vi "GHV232 CRAB Error Message.vi"(11 "Receive Packet":string) -> (0 "Message":string)   [LabVIEW 2017]
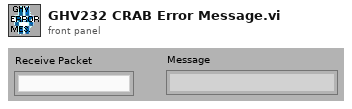
[diagram p1: front panel]
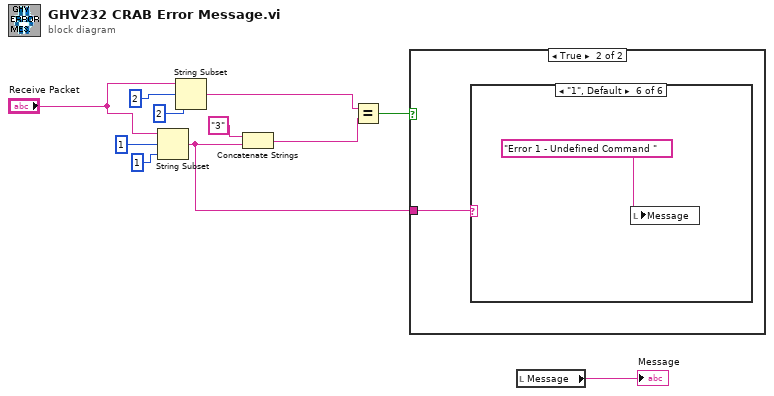
[diagram p0: block diagram]
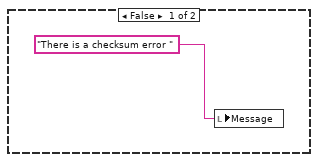
[diagram p2: hidden frame]
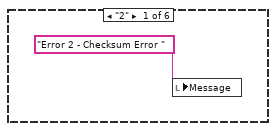
[diagram p3: hidden frame]
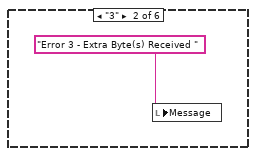
[diagram p4: hidden frame]
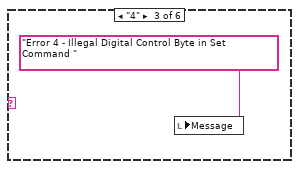
[diagram p5: hidden frame]
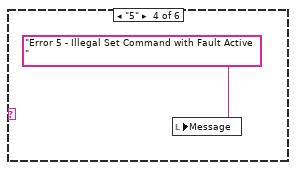
[diagram p6: hidden frame]
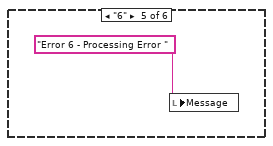
[diagram p7: hidden frame]
diagram:
  n1 = String Subset(string="Receive Packet", offset (0)=1, length (rest)=1) -> (substring=w5:string)
  n2 = String Subset(string="Receive Packet", offset (0)=2, length (rest)=2) -> (substring=w3:string)
  n3 = Concatenate Strings("3", w5) -> (w2:string)
  n4 = Equal?(x=w3, y=w2) -> (x = y?=w7:bool)
  n5 = case shown="True" w7 {
    tunnel: w5 -> [_ w13]
    frame False {
      n6 = local write "Message"("There is a checksum error ") -> ()
    }
    frame True {
      n7 = case shown="\"1\", Default" w13 {
        frame "2" {
          n8 = local write "Message"("Error 2 - Checksum Error ") -> ()
        }
        frame "3" {
          n9 = local write "Message"("Error 3 - Extra Byte(s) Received ") -> ()
        }
        frame "4" {
          n10 = local write "Message"("Error 4 - Illegal Digital Control Byte in Set Command ") -> ()
        }
        frame "5" {
          n11 = local write "Message"("Error 5 - Illegal Set Command with Fault Active ") -> ()
        }
        frame "6" {
          n12 = local write "Message"("Error 6 - Processing Error ") -> ()
        }
        frame "1", Default {
          n13 = local write "Message"("Error 1 - Undefined Command ") -> ()
        }
      }
    }
  }
  n14 = local read "Message"() -> (→"Message":string)
